vi "Curriculum Launcher.vi"(5 "Array of VISA Resources":refnum<visa-resource-name>[](array[refnum]), 7 "Device type":string[](array[string]), 8 "error in (no error)":errorcluster, 10 "Is the required hardware detected?":bool[](array[boolean]), 11 "Example File Paths":path[](array[path])) -> (0 "error out":errorcluster)   [LabVIEW 2020]
panel:
  in  "Multicolumn Listbox":i32(listbox)
  in  "Open Excercise Manual":bool
  in  "Open Button":bool
  # "If hardware is detected, the device references will be \npassed to the example."
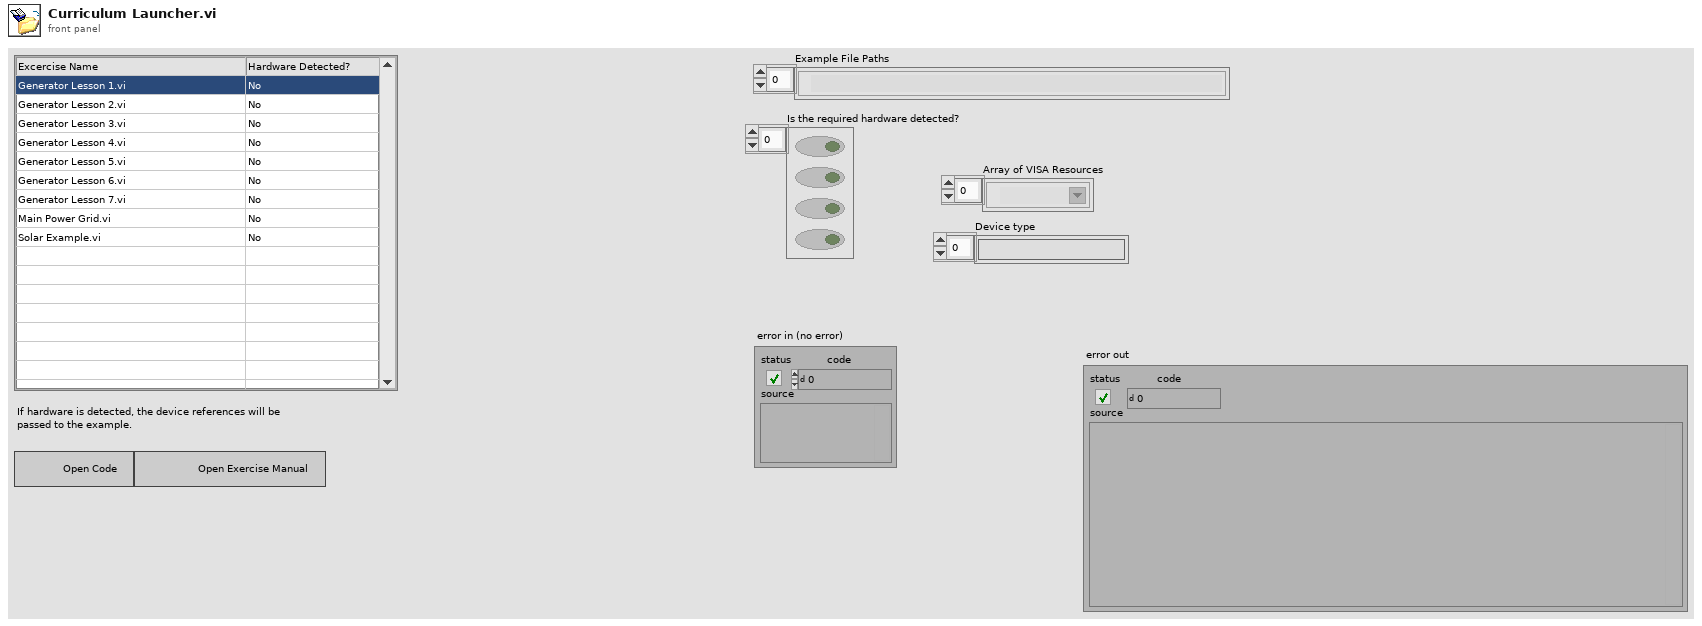
[diagram p1: front panel]
types:
  T1 = enum8{"Enabled", "Disabled", "Disabled and Grayed Out"}
  T2 = cluster{"Open Button":refnum<vi>, "Open Excercise Manual":refnum<vi>}
  T3 = enum32{"Invalid", "Standard", "Closed", "Hidden", "Minimized", "Maximized"}
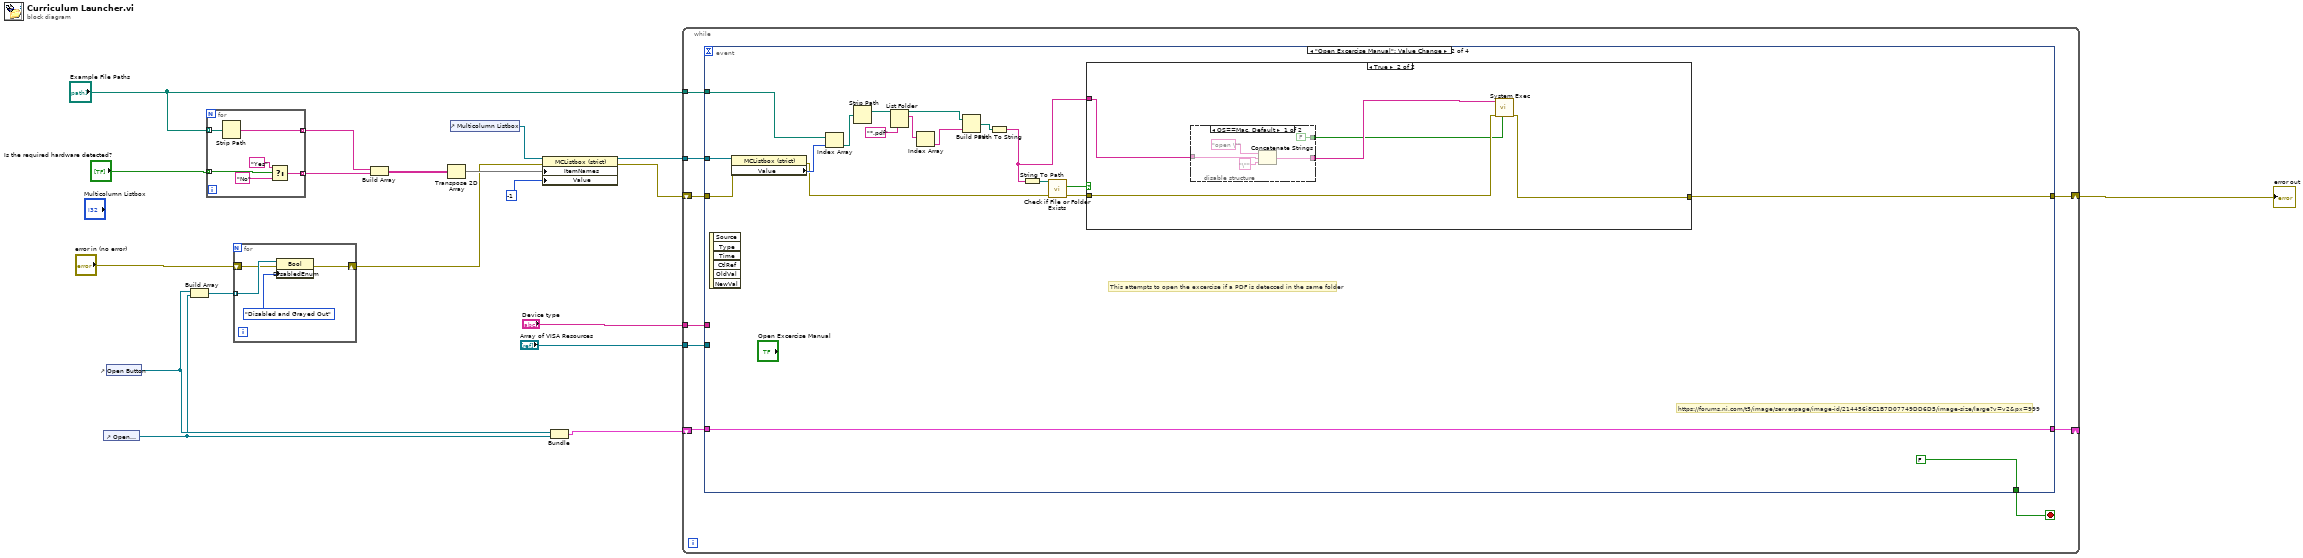
[diagram p0: block diagram]
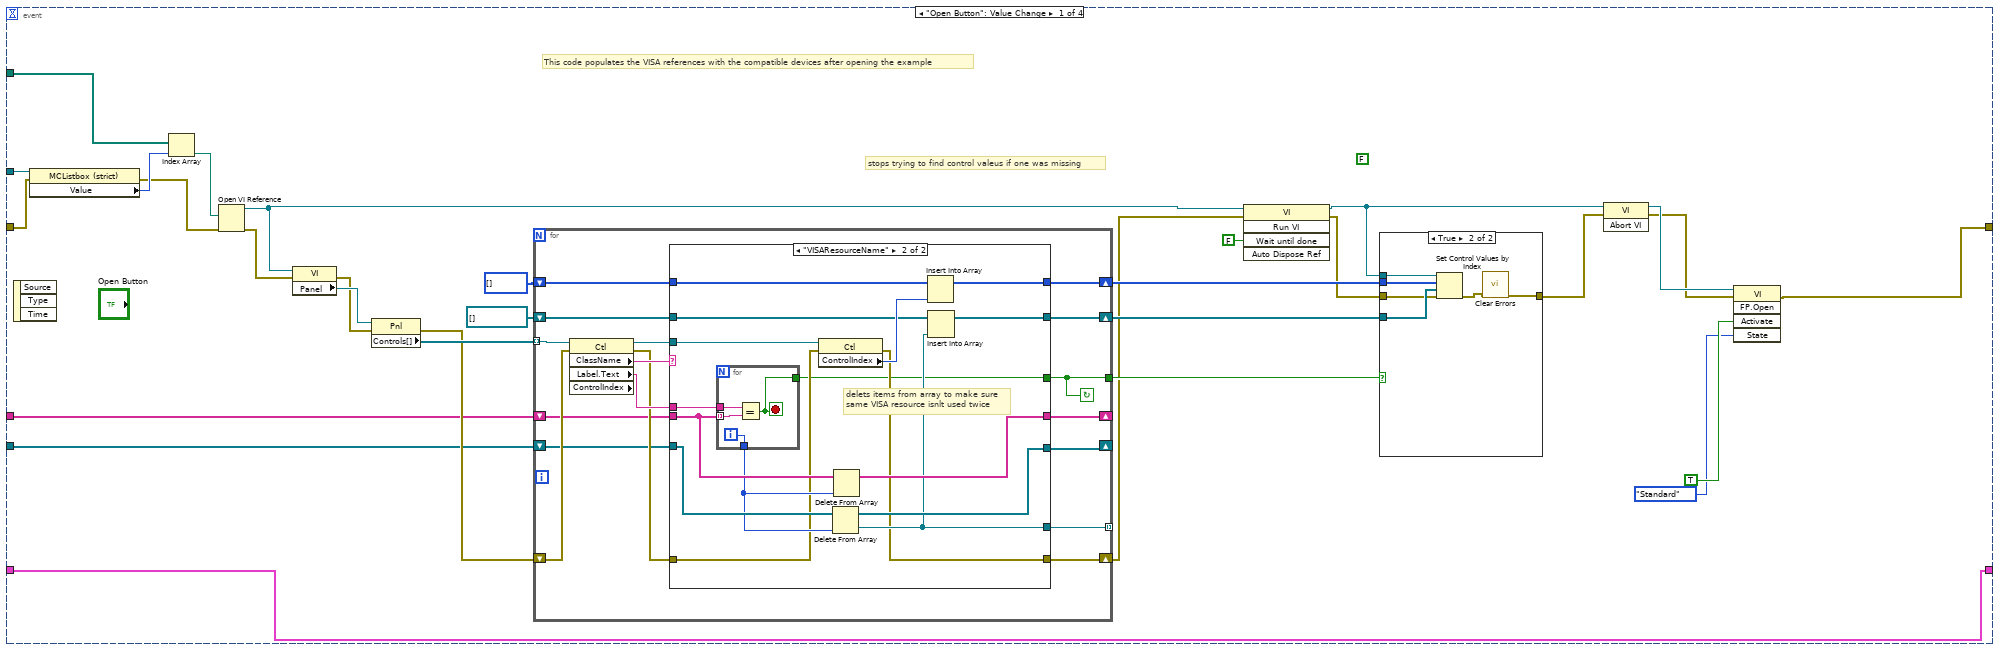
[diagram p2: hidden frame]
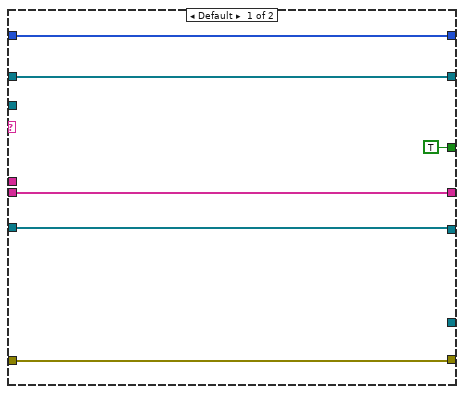
[diagram p4: hidden frame]
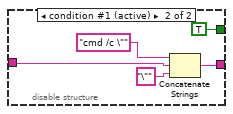
[diagram p6: hidden frame]
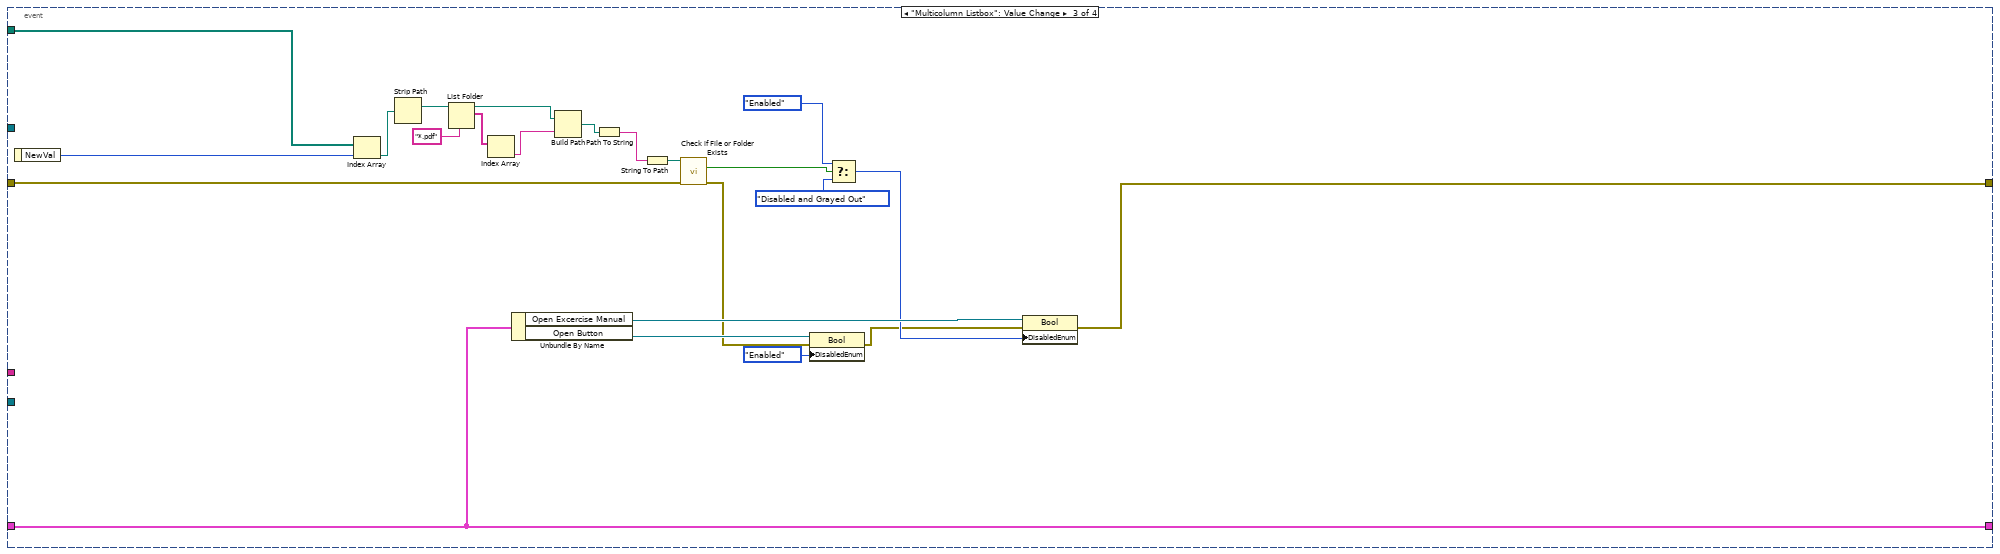
[diagram p7: hidden frame]
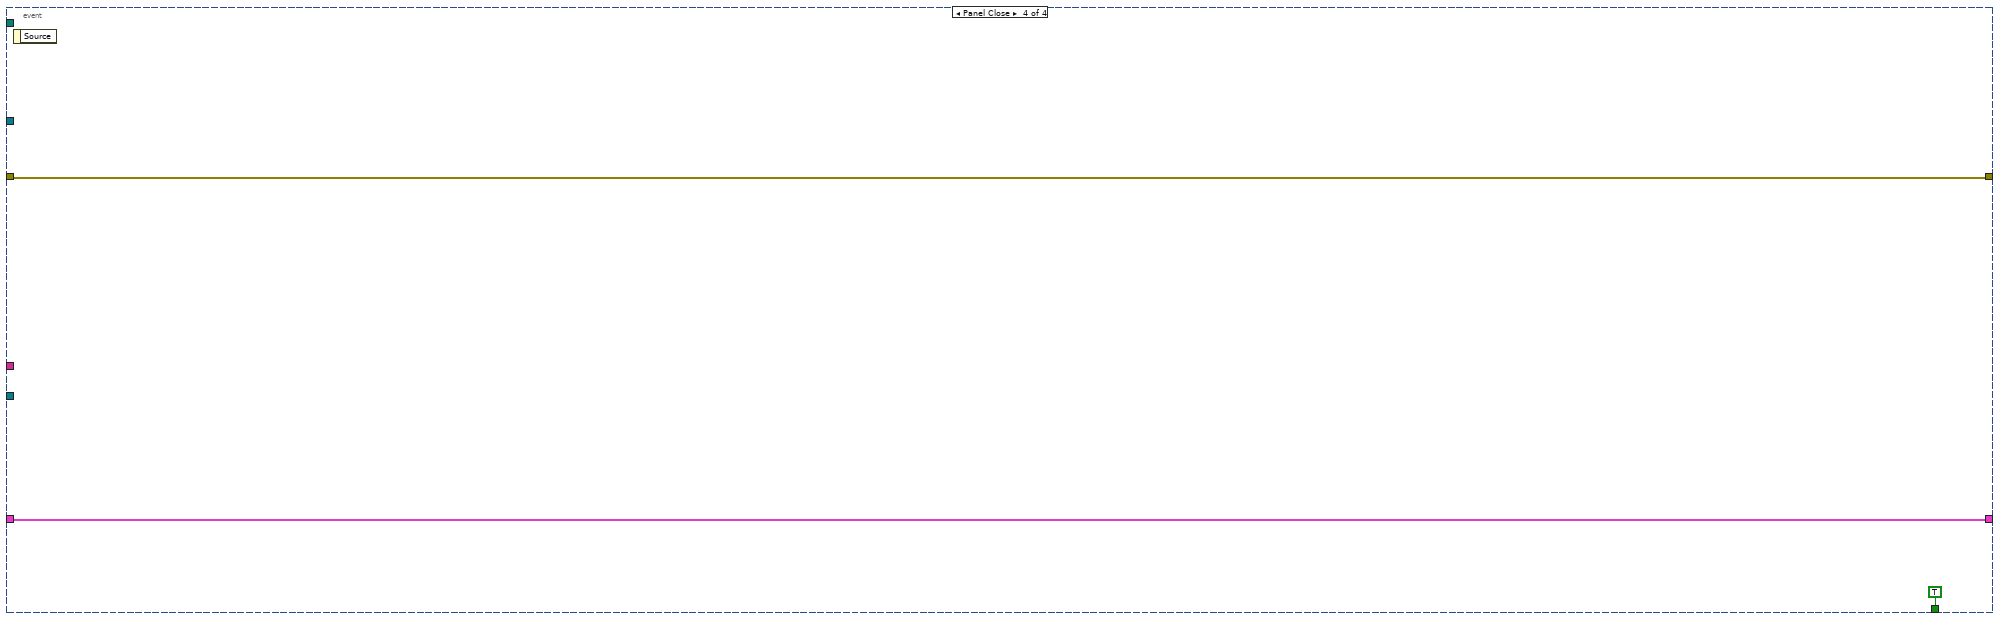
[diagram p8: hidden frame]
diagram:
  n1 = control-ref of="Open Excercise Manual"() -> (w12:refnum<vi>)
  n2 = control-ref of="Open Button"() -> (w13:refnum<vi>)
  n3 = Build Array(w13, w12) -> (w11:refnum<vi>[])
  n4 = for {
    tunnel: "Example File Paths" -> [w25] mode=indexing
    tunnel: [w20] -> w8 mode=indexing
    tunnel: "Is the required hardware detected?" -> [w24] mode=indexing
    tunnel: [w21] -> w7 mode=indexing
    n5 = Strip Path(path=w25) -> (name=w20:string)  [unwired: 1 out]
    n6 = Select(t="Yes" ("concatenated string"), s=w24, f="No" ("concatenated string")) -> (s? t:f=w21:string)
  }
  n7 = for {
    tunnel: w11 -> [w28] mode=indexing
    shift-right: [w26] -> w1
    shift-left: "error in (no error)" -> [w27]
    n8 = property class="Bool"(reference=w28, error in=w27, "DisabledEnum"=T1."Disabled and Grayed Out" ("Disabled")) -> (error out=w26:errorcluster)  [unwired: 1 out]
  }
  n9 = Build Array(w8, w7) -> (w5:string[][])
  n10 = Transpose 2D Array(2D array=w5) -> (transposed array=w4:string[][])
  n11 = control-ref of="Multicolumn Listbox"() -> (w9:refnum<vi>)
  n12 = property on="Property Node" class="MCListbox (strict)"(reference=w9, error in=w1, "ItemNames"=w4, "Value"=-1) -> (reference out=w3:refnum<vi>, error out=w2:errorcluster)
  n13 = Bundle("Open Button"=w13, "Open Excercise Manual"=w12) -> (w14:T2)  [unwired: 1 in]
  n14 = while {
    tunnel: w3 -> [w37]
    tunnel: "Example File Paths" -> [w36]
    shift-right: [w35] -> w15
    shift-left: w2 -> [w38]
    tunnel: "Array of VISA Resources" -> [w34]
    tunnel: "Device type" -> [w33]
    shift-right: [w30] -> _
    shift-left: w14 -> [w31]
    stop <- w32 stop-if-true
    n15 = event shown="[1] \"Open Excercise Manual\": Value Change" {
      selector: _ -> [_ _ _ _]
      dyn-events: _ -> [_ _ _ _]
      timeout: _ -> [_ _ _ _]
      tunnel: w38 -> [w64 w132 w162 w179]
      tunnel: w37 -> [w68 w134 _ _]
      tunnel: w36 -> [w66 w133 w164 _]
      tunnel: [w41 w137 w154 w179] -> w35
      tunnel: w34 -> [w57 _ _ _]
      tunnel: w33 -> [w56 _ _ _]
      tunnel: [_ FALSE _ TRUE] -> w32
      tunnel: w31 -> [w50 w119 w174 w177]
      tunnel: [w50 w119 w174 w177] -> w30
      event "Open Button": Value Change {
        (unwired) FALSE ("Wait Until Done")
        # "This code populates the VISA references with the compatible devices after opening the example"
        # "stops trying to find control valeus if one was missing"
        n16 = event-data() -> ()  [unwired: 1 in, 3 out]
        n17 = property on="Property Node" class="MCListbox (strict)"(reference=w68, error in=w64) -> (error out=w63:errorcluster, "Value"=w67:i32)  [unwired: 1 out]
        n18 = Index Array(array=w66, index=w67) -> (element=w65:path)
        n19 = Open VI Reference(vi path=w65, error in (no error)=w63) -> (vi reference=w48:refnum<vi>, error out=w58:errorcluster)  [unwired: 4 in]
        n20 = property class="VI"(reference=w48, error in=w58) -> (error out=w60:errorcluster, "Panel"=w62:refnum<vi>)  [unwired: 1 out]
        n21 = property class="Pnl"(reference=w62, error in=w60) -> (error out=w59:errorcluster, "Controls[]"=w61:refnum<vi>[])  [unwired: 1 out]
        n22 = for {
          tunnel: w61 -> [w92] mode=indexing
          shift-right: [w87] -> w39
          shift-left: w59 -> [w90]
          shift-right: [w84] -> _
          shift-left: w56 -> [w85]
          shift-right: [w83] -> _
          shift-left: w57 -> [w86]
          tunnel: [w82] -> _ mode=indexing
          shift-right: [w80] -> w52
          shift-left: refnum<visa-resource-name>[] [] -> [w77]
          shift-right: [w79] -> w53
          shift-left: i32[] [] -> [w78]
          tunnel: [w76] -> w51
          stop <- w76 continue-if-true
          n23 = property class="Ctl" props=["ClassName", "Label", "Text", "ControlIndex"](reference=w92, error in=w90) -> (reference out=w81:refnum<vi>, error out=w88:errorcluster, "ClassName"=w91:string, "Label.Text"=w89:string)  [unwired: 1 out]
          n24 = case shown="\"VISAResourceName\"" w91 {
            tunnel: w89 -> [_ w114]
            tunnel: w88 -> [w96 w107]
            tunnel: [w96 w100] -> w87
            tunnel: w86 -> [w97 w113]
            tunnel: w85 -> [w98 w112]
            tunnel: [w98 w110] -> w84
            tunnel: [w97 w109] -> w83
            tunnel: [_ w105] -> w82
            tunnel: w81 -> [_ w108]
            tunnel: [w94 w104] -> w80
            tunnel: [w95 w103] -> w79
            tunnel: w78 -> [w95 w102]
            tunnel: w77 -> [w94 w101]
            tunnel: [TRUE w99] -> w76
            frame Default {
            }
            frame "VISAResourceName" {
              # "delets items from array to make sure\nsame VISA resource isnlt used twice"
              n25 = for {
                tunnel: w114 -> [w118]
                tunnel: w112 -> [w117] mode=indexing
                tunnel: [w116] -> w111
                tunnel: [w115] -> w99
                i -> [w116]
                stop <- w115 stop-if-true
                n26 = Equal?(x=w118, y=w117) -> (x = y?=w115:bool)
              }
              n27 = property class="Ctl"(reference=w108, error in=w107) -> (error out=w100:errorcluster, "ControlIndex"=w106:i32)  [unwired: 1 out]
              n28 = Delete From Array(array=w113, index=w111) -> (deleted portion=w105:refnum<visa-resource-name>, array with subset deleted=w109:refnum<visa-resource-name>[])  [unwired: 1 in]
              n29 = Delete From Array(array=w112, index=w111) -> (array with subset deleted=w110:string[])  [unwired: 1 in, 1 out]
              n30 = Insert Into Array(array=w102, new element=w106) -> (w103:i32[])  [unwired: 1 in]
              n31 = Insert Into Array(array=w101, new element=w105) -> (w104:refnum<visa-resource-name>[])  [unwired: 1 in]
            }
          }
        }
        n32 = invoke class="VI" method="Run VI"(reference=w48, error in=w39, "Wait until done"=FALSE ("Wait Until Done")) -> (reference out=w46:refnum<vi>, error out=w40:errorcluster)  [unwired: 2 in, 3 out]
        n33 = case shown="True" w51 {
          tunnel: w53 -> [_ w75]
          tunnel: w52 -> [_ w74]
          tunnel: [w69 w70] -> w47
          tunnel: w46 -> [_ w73]
          tunnel: w40 -> [w69 w72]
          frame False {
          }
          frame True {
            n34 = Set Control Values by Index(0:w73, 1:w75, 2:w74, 3:w72) -> (11:w71:errorcluster)
            n35 = call <vilib>:"Clear Errors.vi"("error in (no error)"=w71) -> ("error out"=w70:errorcluster)  [unwired: 5 in, 1 out]
          }
        }
        n36 = invoke class="VI" method="Abort VI"(reference=w46, error in=w47) -> (reference out=w45:refnum<vi>, error out=w42:errorcluster)  [unwired: 1 in, 1 out]
        n37 = invoke class="VI" method="FP.Open"(reference=w45, error in=w42, "Activate"=TRUE ("Activate?"), "State"=T3."Standard") -> (error out=w41:errorcluster)  [unwired: 1 in, 4 out]
      }
      event "Open Excercise Manual": Value Change {
        # "https://forums.ni.com/t5/image/serverpage/image-id/214456i8C1B7D07749DD6D5/image-size/large?v=v2&px=999"
        # "This attempts to open the excercise if a PDF is detecced in the same folder"
        n38 = event-data() -> ()  [unwired: 1 in, 6 out]
        n39 = property on="Property Node" class="MCListbox (strict)"(reference=w134, error in=w132) -> (error out=w129:errorcluster, "Value"=w135:i32)  [unwired: 1 out]
        n40 = Index Array(array=w133, index=w135) -> (element=w127:path)
        n41 = Strip Path(path=w127) -> (stripped path=w126:path)  [unwired: 1 out]
        n42 = List Folder(path=w126, pattern="*.pdf") -> (path out=w123:path, filenames=w124:string[])  [unwired: 2 in, 2 out]
        n43 = Index Array(array=w124) -> (element=w122:string)  [unwired: 1 in]
        n44 = Build Path(base path=w123, name or relative path=w122) -> (appended path=w121:path)
        n45 = Path To String(path=w121) -> (string=w120:string)
        n46 = String To Path(string=w120) -> (path=w131:path)
        n47 = call <vilib>:"Check if File or Folder Exists.vi"("error in (no error)"=w129, "path"=w131) -> ("error out"=w128:errorcluster, "file or folder exists?"=w130:bool)  [unwired: 7 in, 1 out]
        n48 = case shown="True" w130 {
          tunnel: [w138 w143] -> w137
          tunnel: w120 -> [_ w141]
          tunnel: w128 -> [w138 w142]
          frame False {
          }
          frame True {
            n49 = disable-structure shown="OS==Mac, Default" {
              disable-tunnel: w141 -> [w146 w151]
              disable-tunnel: [w145 w150] -> w140
              disable-tunnel: [FALSE ("run minimized? (F)") TRUE ("run minimized? (F)")] -> w139
              frame condition #0 {
                n50 = Concatenate Strings("open \"" ("string"), w146, "\"" ("string")) -> (w145:string)
              }
              frame condition #1 (active) {
                n51 = Concatenate Strings("cmd /c \"" ("string"), w151, "\"" ("string")) -> (w150:string)
              }
            }
            n52 = call <vilib>:"System Exec.vi"("run minimized? (F)"=w139, "error in (no error)"=w142, "command line"=w140) -> ("error out"=w143:errorcluster)  [unwired: 5 in, 3 out]
          }
        }
      }
      event "Multicolumn Listbox": Value Change {
        n53 = event-data() -> ("NewVal"=w163:i32)  [unwired: 1 in]
        n54 = Index Array(array=w164, index=w163) -> (element=w172:path)
        n55 = Strip Path(path=w172) -> (stripped path=w171:path)  [unwired: 1 out]
        n56 = List Folder(path=w171, pattern="*.pdf") -> (path out=w168:path, filenames=w169:string[])  [unwired: 2 in, 2 out]
        n57 = Index Array(array=w169) -> (element=w167:string)  [unwired: 1 in]
        n58 = Unbundle By Name(w174) -> ("Open Excercise Manual"=w161:refnum<vi>, "Open Button"=w176:refnum<vi>)
        n59 = Build Path(base path=w168, name or relative path=w167) -> (appended path=w166:path)
        n60 = Path To String(path=w166) -> (string=w165:string)
        n61 = String To Path(string=w165) -> (path=w173:path)
        n62 = call <vilib>:"Check if File or Folder Exists.vi"("error in (no error)"=w162, "path"=w173) -> ("error out"=w156:errorcluster, "file or folder exists?"=w160:bool)  [unwired: 7 in, 1 out]
        n63 = property class="Bool"(reference=w176, error in=w156, "DisabledEnum"=T1."Enabled" ("Disabled")) -> (error out=w155:errorcluster)  [unwired: 1 out]
        n64 = Select(t=T1."Enabled" ("Disabled"), s=w160, f=T1."Disabled and Grayed Out" ("Disabled")) -> (s? t:f=w157:T1)
        n65 = property class="Bool"(reference=w161, error in=w155, "DisabledEnum"=w157) -> (error out=w154:errorcluster)  [unwired: 1 out]
      }
      event Panel Close {
        n66 = event-data() -> ()  [unwired: 1 in, 1 out]
      }
    }
  }
  "error out" <- w15
